vi "Write DAC.vi"(8 "error in (no error)":errorcluster, 10 "Analog Output":u16, 11 "I2C_0-20mA(GP8313) in":refnum<class "I2C_0-20mA(GP8313).lvclass">) -> (0 "error out":errorcluster, 3 "I2C_0-20mA(GP8313) out":refnum<class "I2C_0-20mA(GP8313).lvclass">)   [LabVIEW 2020, in "CTI-Peripheral.lvlib" / "I2C_0-20mA(GP8313).lvclass"]
uses:
  I2C_0-20mA(GP8313).lvclass
  I2C_0-20mA(GP8313).lvclass/I2C_0-20mA(GP8313).ctl
  CTI/I2C Connection/I2C Connection.lvclass/I2C Connection.ctl
  CTI/Session/I2C Write Data.vi
  CTI/I2C Connection/I2C Connection.lvclass
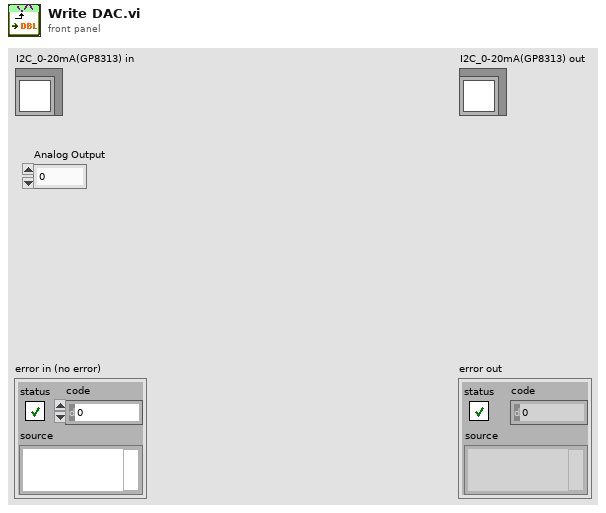
[diagram p1: front panel]
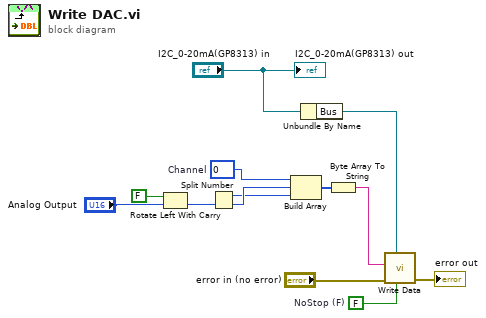
[diagram p0: block diagram]
diagram:
  w9 = u8 0  # Channel
  w10 = FALSE  # NoStop (F)
  n1 = Rotate Left With Carry(2:"Analog Output", 3:FALSE ("carry")) -> (0:w7:u16)  [unwired: 1 out]
  n2 = Split Number(x=w7) -> (hi(x)=w5:u8, lo(x)=w6:u8)
  n3 = Build Array(w9, w6, w5) -> (w4:u8[])
  n4 = Unbundle By Name("I2C_0-20mA(GP8313) in") -> ("Bus"=w11:refnum<class "I2C Connection.lvclass">)
  n5 = Byte Array To String(unsigned byte array=w4) -> (string=w1:string)
  n6 = call "Write Data.vi"("NoStop (F)"=w10, "I2C Connection"=w11, "error in (no error)"="error in (no error)", "Data"=w1) -> ("error out"=→"error out":errorcluster)  [unwired: 7 in]
  "I2C_0-20mA(GP8313) out" <- "I2C_0-20mA(GP8313) in"
